vi "Phasor Compute Gated Decay (Fixed Integration Steps).vi"(4 "Non Dirac IRF or non-0 lifetime":bool, 6 "# Steps":i32, 8 "Error In":errorcluster, 9 "IRF Period":dbl, 10 "Gate & Decay Parameters Array":T1[](array[typedef]) {"A" format="%#_4g"; "s" format="%#_4g"; "sF" format="%#_4g"; "sR" format="%#_4g"; "t_i" format="%#_4g"; "t_0" format="%#_4g"; "tau" format="%#_4g"; "T" format="%#_4g"; "W" format="%#_4g"}, 11 "Time Points {t_i}":dbl[](array[numeric])) -> (0 "Error Out":errorcluster, 3 "{F(t_i)}":dbl[](array[numeric]))   [LabVIEW 2021, in "Phasor.lvlib"]
uses:
  Phasor.lvlib
  Phasor Gate & Decay Parameters.ctl
  Phasor Gate Type.ctl
  Phasor IRF Model.ctl
  Graphs/XY Graph/XY Plot Data.ctl
  Phasor Compute Gate-IRF Array.vi
  Graphs/XY Graph/XY Graph Interpolate Plot at x.vi
  Phasor Compute Gate-IRF Array.vi/7d9bb666-8e44-4efd-bf11-38a816117c5c.vi
  Phasor Abort Parallel Computation.vi
  Math/T-Periodic Square Gate.vi
  Math/T-Periodic Triangle Gate.vi
  Math/T-Periodic Sawtooth Gate.vi
  <vilib>/Utility/error.llb/Error Cluster From Error Code.vi
  Math/T-Periodic Finite Edge Square Gate.vi
  Math/T-Periodic Finite Edge Tilted Top Square Gate.vi
  Phasor Compute 1-Exp Array.vi
  <vilib>/ErrorRing/Error Ring.xnode
  <vilib>/Analysis/2dsp.llb/Integral Method.ctl
  <vilib>/Analysis/NI_AALPro.lvlib
  Error/Error.lvlib
  <vilib>/Analysis/8numeric.llb/1D Numeric Integration.vi
  Utilities/Utilities.lvlib
  Fits/Fits.lvlib
  Graphs/XY Graph/XY Graph Add-Ons.lvlib
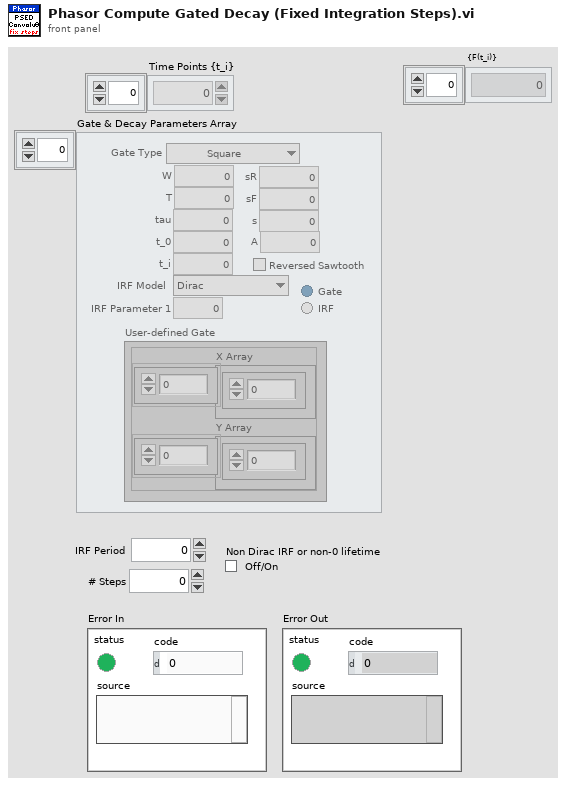
[diagram p1: front panel]
types:
  T1 = typedef "Phasor.lvlib/Phasor Gate & Decay Parameters.ctl" = cluster{"W":dbl, "T":dbl, "tau":dbl, "t_0":dbl, "Gate Type":T2, "t_i":dbl, "sR":dbl, "sF":dbl, "s":dbl, "Reversed Sawtooth":bool, "IRF Model":T3, "IRF Parameter 1":dbl, "User-defined Gate":T4, "Type of User-defined Function":enum32{"Gate", "IRF"}, "A":dbl}
  T2 = typedef "Phasor.lvlib/Phasor Gate Type.ctl" = enum16{"Square", "Finite Edge Square", "Finite Edge, Tilted Top Square", "Triangle", "Sawtooth", "User-defined"}
  T3 = typedef "Phasor.lvlib/Phasor IRF Model.ctl" = enum16{"Dirac", "Exponential"}
  T4 = typedef "XY Graph Add-Ons.lvlib/XY Plot Data.ctl" = cluster{"X Array":dbl[], "Y Array":dbl[]}
  T5 = typedef "NI_AALPro.lvlib/Integral Method.ctl" = i32
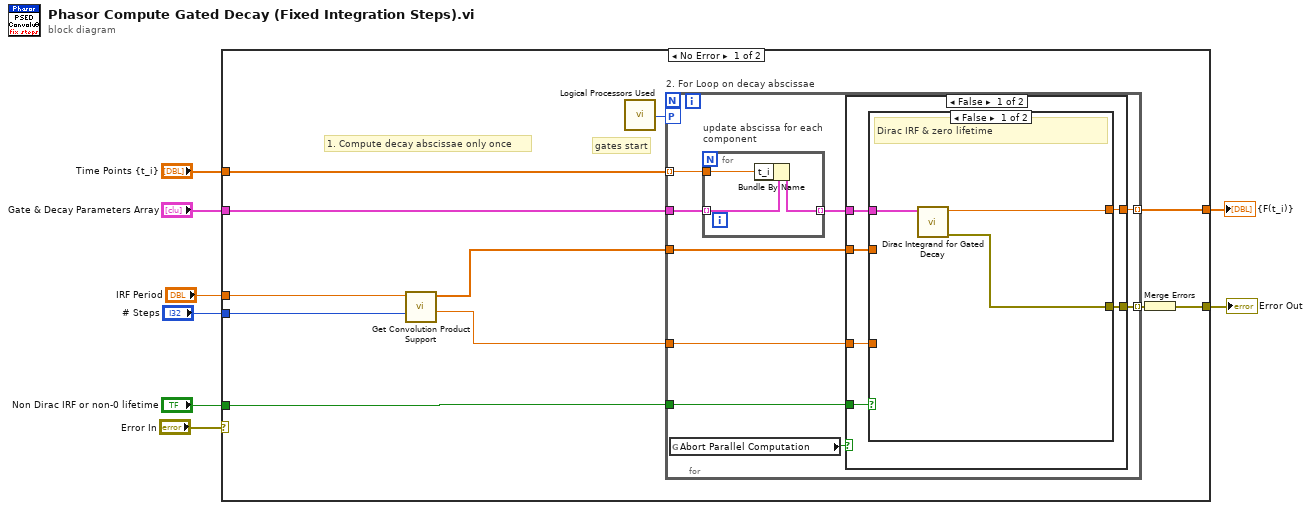
[diagram p0: block diagram]
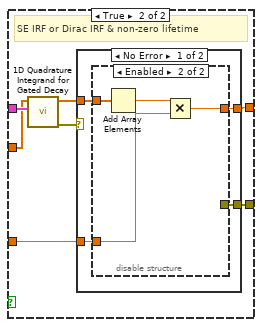
[diagram p2: hidden frame]
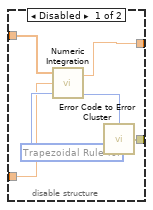
[diagram p3: hidden frame]
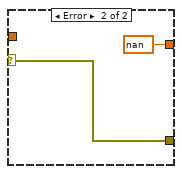
[diagram p4: hidden frame]
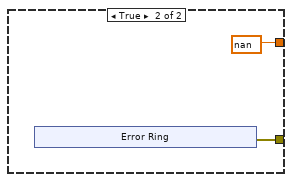
[diagram p5: hidden frame]
diagram:
  n1 = case shown="No Error" "Error In" {
    selector: "Error In" -> [_ w70]
    tunnel: "Non Dirac IRF or non-0 lifetime" -> [w19 _]
    tunnel: "IRF Period" -> [w18 _]
    tunnel: "# Steps" -> [w10 _]
    tunnel: "Time Points {t_i}" -> [w16 _]
    tunnel: "Gate & Decay Parameters Array" -> [w14 _]
    tunnel: [w13 _] -> w3
    tunnel: [w12 w70] -> w2
    frame No Error {
      # "1. Compute decay abscissae only once"
      # "gates start"
      n2 = call "Get Convolution Product Support.vi"("# Values"=w10, "IRF Period"=w18) -> ("Step"=w9:dbl, "Ramp"=w15:dbl[])  [unwired: 7 in, 1 out]
      n3 = call "Logical Processors Used.vi"() -> ("# Logical Processor Used"=w11:i32)  [unwired: 6 in]
      n4 = for "2. For Loop on decay abscissae" {
        tunnel: w14 -> [w28]
        tunnel: w16 -> [w22] mode=indexing
        tunnel: w15 -> [w26]
        tunnel: [w25] -> w13 mode=indexing
        tunnel: w9 -> [w24]
        workers-P: w11 -> [_]
        tunnel: [w23] -> w17 mode=indexing
        tunnel: w19 -> [w21]
        n5 = global read "Phasor Abort Parallel Computation.vi" "Abort Parallel Computation"() -> (w20:bool)
        n6 = for "update abscissa for each component" {
          tunnel: w28 -> [w31] mode=indexing
          tunnel: [w30] -> w27 mode=indexing
          tunnel: w22 -> [w29]
          n7 = Bundle By Name(cluster=w31, "t_i"=w29) -> (w30:T1)
        }
        n8 = case shown="False" w20 {
          tunnel: w27 -> [w37 _]
          tunnel: w26 -> [w36 _]
          tunnel: [w35 nan ("result")] -> w25
          tunnel: w24 -> [w34 _]
          tunnel: [w33 w64] -> w23
          tunnel: w21 -> [w32 _]
          frame False {
            n9 = case shown="False" w32 {
              tunnel: w37 -> [w40 w47]
              tunnel: w36 -> [_ w45]
              tunnel: [w39 w44] -> w35
              tunnel: w34 -> [_ w43]
              tunnel: [w38 w41] -> w33
              frame False {
                # "Dirac IRF & zero lifetime"
                n10 = call "Dirac Integrand for Gated Decay.vi"("data"=w40) -> ("Error Out"=w38:errorcluster, "F(X)"=w39:dbl)  [unwired: 9 in]
              }
              frame True {
                # "SE IRF or Dirac IRF & non-zero lifetime"
                n11 = call "1D Quadrature Integrand for Gated Decay.vi"("data"=w47, "X"=w45) -> ("Error Out"=w42:errorcluster, "F(X)"=w46:dbl[])  [unwired: 8 in]
                n12 = case shown="No Error" w42 {
                  selector: w42 -> [_ w63]
                  tunnel: w46 -> [w51 _]
                  tunnel: [w50 nan ("result")] -> w44
                  tunnel: w43 -> [w49 _]
                  tunnel: [w48 w63] -> w41
                  frame No Error {
                    n13 = disable-structure shown="Enabled" {
                      disable-tunnel: w51 -> [w56 w61]
                      disable-tunnel: [w55 w58] -> w50
                      disable-tunnel: w49 -> [w54 w59]
                      disable-tunnel: [w52 _] -> w48
                      frame Disabled {
                        w57 = T5 0 items=["Trapezoidal Rule", "Simpson's Rule", "Simpson's 3/8 Rule", "Bode Rule"] ("integration method")
                        n14 = call-poly <vilib>:"Numeric Integration.vi"("integration method"=w57, "dt"=w54, "Input Array"=w56) -> ("error"=w53:i32, "result"=w55:dbl)
                        n15 = call "Error Code to Error Cluster.vi"("Error Code"=w53) -> ("Error Out"=w52:errorcluster)  [unwired: 14 in]
                      }
                      frame Enabled {
                        n16 = Add Array Elements(numeric array=w61) -> (sum=w60:dbl)
                        n17 = Multiply(x=w60, y=w59) -> (x*y=w58:dbl)
                      }
                    }
                  }
                  frame Error {
                  }
                }
              }
            }
          }
          frame True {
            n18 = xnode "Error Ring"() -> ("error out"=w64:errorcluster)
          }
        }
      }
      n19 = Merge Errors(w17) -> (w12:errorcluster)
    }
    frame Error {
    }
  }
  "{F(t_i)}" <- w3
  "Error Out" <- w2
